vi "set_immersion.vi"(8 "error in (no error)":errorcluster, 10 "Immersion":T1, 11 "GenericObjective in":refnum<class "GenericObjective.lvclass">) -> (0 "error out":errorcluster, 3 "GenericObjective out":refnum<class "GenericObjective.lvclass">)   [LabVIEW 2010, in "GenericObjective.lvclass"]
uses:
  GenericObjective.lvclass
  immersion_enum.ctl
  GenericObjective.lvclass/GenericObjective.ctl
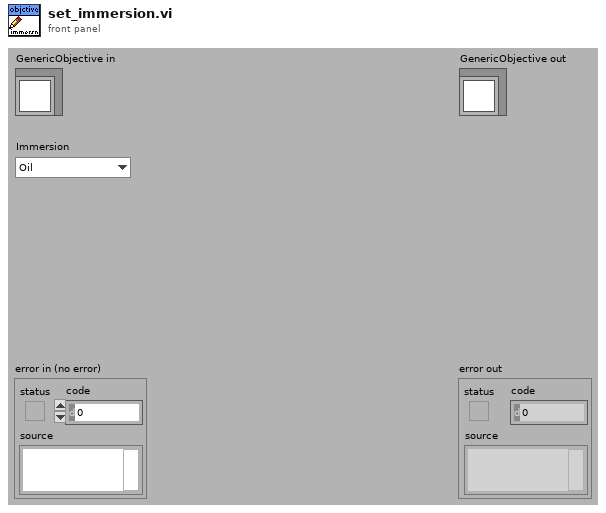
[diagram p1: front panel]
types:
  T1 = typedef "GenericObjective.lvclass/immersion_enum.ctl" = enum16{"Oil", "Water", "WaterDipping", "Air", "Multi", "Glycerol", "Other", "Unknown"}
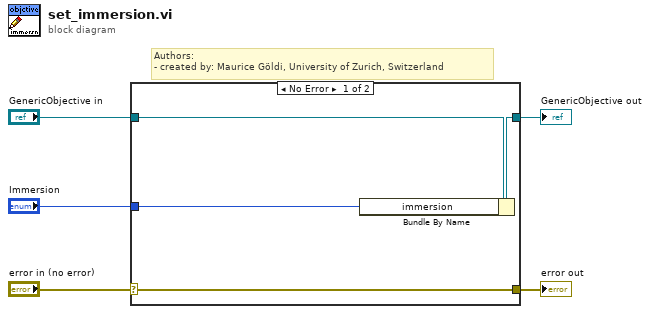
[diagram p0: block diagram]
diagram:
  # "Authors: \n- created by: Maurice Göldi, University of Zurich, Switzerland"
  n1 = case shown="No Error" "error in (no error)" {
    selector: "error in (no error)" -> [w9 w10]
    tunnel: [w9 w10] -> w4
    tunnel: [w7 w11] -> w2
    tunnel: "GenericObjective in" -> [w8 w11]
    tunnel: "Immersion" -> [w6 _]
    frame No Error {
      n2 = Bundle By Name(cluster=w8, "immersion"=w6) -> (w7:refnum<class "GenericObjective.lvclass">)
    }
    frame Error {
    }
  }
  "error out" <- w4
  "GenericObjective out" <- w2
